vi "CT_AddHallProbeOntoFastFire.vi"(0 "task in":refnum<k21>="PCIE-FastFire", 5 "Chan Delays":dbl[](array[numeric])=[0.0001, 0.0003, 0.0005, 0.0007, 0.0013] format="%.6f", 7 "CT Fast Fire":digitalwaveform[](graph), 9 "Enable Channel":bool, 11 "error in":errorcluster) -> (4 "task out":refnum<k21>, 8 "Digital Waveform Graph":digitalwaveform[](graph), 15 "error out":errorcluster)   [LabVIEW 2009]
doc: "This subVI creates an N dimensional Boolean array based on the number of channels in the task."
uses:
  <vilib>/Waveform/DWDTOps.llb/DWDT Boolean Array to Digital.vi
  Program Files (x86)/National Instruments/LabVIEW 2009/resource/objmgr/daqmx.rc
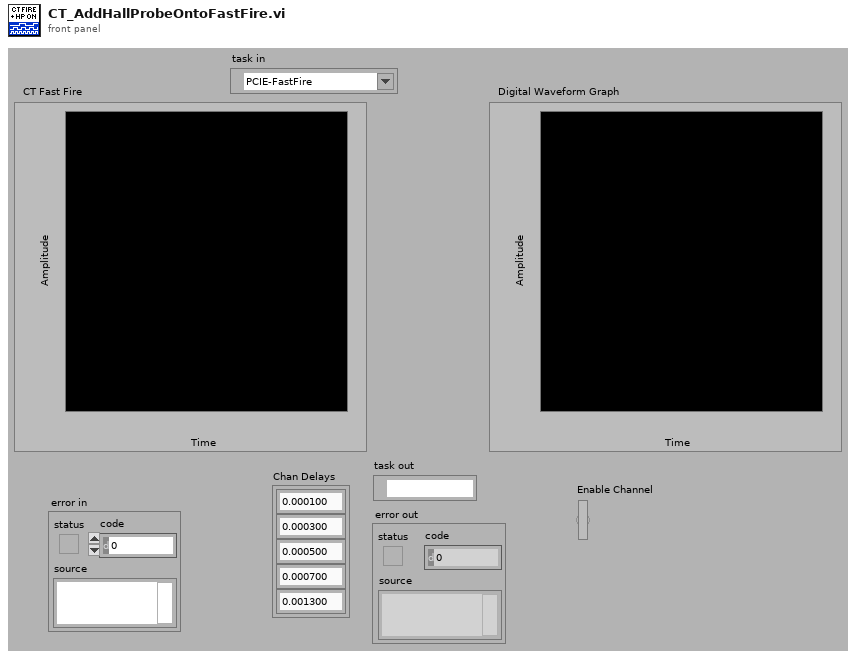
[diagram p1: front panel]
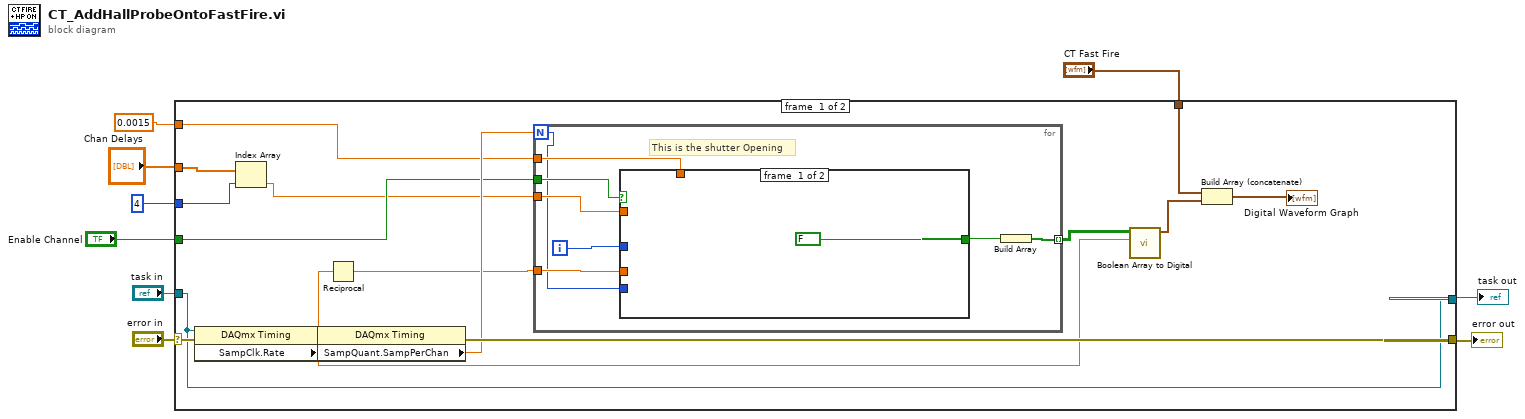
[diagram p0: block diagram]
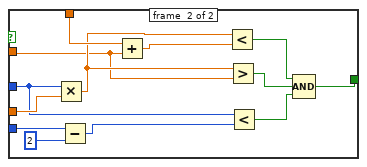
[diagram p2: hidden frame]
diagram:
  n1 = case shown="No Error" "error in" {
    selector: "error in" -> [w26 w49]
    tunnel: "task in" -> [w10 w50]
    tunnel: [w10 w50] -> w8
    tunnel: [w23 w49] -> w6
    tunnel: "Chan Delays" -> [w22 _]
    tunnel: 4 -> [w21 _]
    tunnel: "Enable Channel" -> [w19 _]
    tunnel: 0.0015 -> [w16 _]
    tunnel: "CT Fast Fire" -> [w13 _]
    frame #0 {
      n2 = property class="DAQmx Timing"(reference=w10, error in=w26) -> (reference out=w25:refnum<k21>, error out=w24:errorcluster, "SampClk.Rate"=w14:dbl)
      n3 = Index Array(array=w22, index=w21) -> (element=w17:dbl)
      n4 = property class="DAQmx Timing"(reference=w25, error in=w24) -> (error out=w23:errorcluster, "SampQuant.SampPerChan"=w20:dbl)  [unwired: 1 out]
      n5 = Reciprocal(x=w14) -> (1/x=w18:dbl)
      n6 = for {
        N: w20 -> [w27]
        tunnel: w17 -> [w33]
        tunnel: w18 -> [w34]
        tunnel: [w32] -> w15 mode=indexing
        tunnel: w19 -> [w29]
        tunnel: w16 -> [w28]
        i -> [w31]
        # "This is the shutter Opening"
        n7 = case shown="True" w29 {
          tunnel: w34 -> [_ w48]
          tunnel: w33 -> [_ w36]
          tunnel: w31 -> [_ w41]
          tunnel: [FALSE w47] -> w30
          tunnel: w28 -> [_ w45]
          tunnel: w27 -> [_ w40]
          frame #0 {
          }
          frame #1 {
            n8 = Multiply(x=w41, y=w48) -> (x*y=w43:dbl)
            n9 = Subtract(x=w40, y=2) -> (x-y=w38:i32)
            n10 = Add(x=w45, y=w36) -> (x+y=w42:dbl)
            n11 = Less?(x=w43, y=w42) -> (x < y?=w44:bool)
            n12 = Greater?(x=w43, y=w36) -> (0:w46:bool)
            n13 = Less?(x=w41, y=w38) -> (x < y?=w37:bool)
            n14 = Compound Arithmetic op=AND(w44, w46, w37) -> (w47:bool)
          }
        }
        n15 = Build Array(w30) -> (w32:bool[])
      }
      n16 = call-poly <vilib>:"Boolean Array to Digital.vi"("sample rate"=w14, "boolean array"=w15) -> ("digital waveform"=w12:digitalwaveform)  [unwired: 8 in, 1 out]
      n17 = Build Array (concatenate)(w13, w12) -> (→"Digital Waveform Graph":digitalwaveform[])
    }
    frame #1 {
    }
  }
  "error out" <- w6
  "task out" <- w8
